vi "FRCts20_Backend_ArchiveTeamData.vi"(8 "error in (no error)":errorcluster) -> (0 "error out":errorcluster, 2 "Status?":string)   [LabVIEW 2014, in "FRCts20_Backend_WebMethods.lvlib"]
uses:
  FRCts20_Backend_WebMethods.lvlib
  FRCts20_Backend_FGVOperation.ctl
  FRCts20_Backend_Engine.lvlib
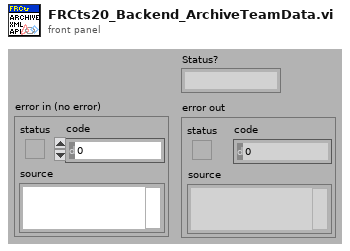
[diagram p1: front panel]
types:
  T1 = typedef "FRCts20_Backend_Engine.lvlib/FRCts20_Backend_FGVOperation.ctl" = enum16{"Initialize", "EnqueueMessage", "EnqueueDataReturn", "FlushMessage", "FlushDataReturn"}
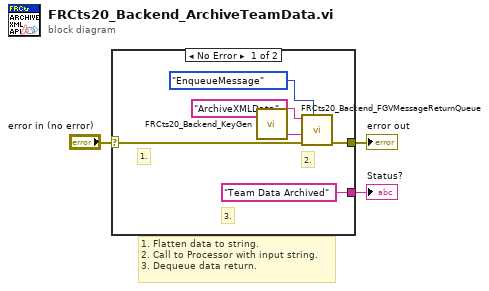
[diagram p0: block diagram]
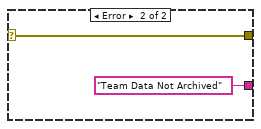
[diagram p2: hidden frame]
diagram:
  # "1. Flatten data to string.\n2. Call to Processor with input string.\n3. Dequeue data return."
  n1 = case shown="No Error" "error in (no error)" {
    selector: "error in (no error)" -> [w6 w11]
    tunnel: [w5 w11] -> w2
    tunnel: ["Team Data Archived" "Team Data Not Archived"] -> w1
    frame No Error {
      # "3."
      # "2."
      # "1."
      n2 = call "FRCts20_Backend_KeyGen.vi"() -> ("Keygen"=w7:string)  [unwired: 27 in]
      n3 = call "FRCts20_Backend_FGVMessageReturnQueue.vi"("Operation"=FRCts20_Backend_FGVOperation."EnqueueMessage", "error in (no error)"=w6, "Key"=w7, "Message Name"="ArchiveXMLData") -> ("error out"=w5:errorcluster)  [unwired: 4 in, 1 out]
    }
    frame Error {
    }
  }
  "error out" <- w2
  "Status?" <- w1
